vi "Set Impulse Data.vi"(8 "error in (no error)":errorcluster, 10 "Impulse Object Reference":T1, 11 "Impulse Manager in":refnum<class "Impulse Manager.lvclass">) -> (0 "error out":errorcluster, 3 "Impulse Manager out":refnum<class "Impulse Manager.lvclass">)   [LabVIEW 2016, in "Impulse Manager.lvclass"]
uses:
  Impulse Manager.lvclass
  Impulse Data/Instance handle.ctl
  Impulse Data/Impulse Data.lvclass
  Impulse Manager.lvclass/Impulse Manager.ctl
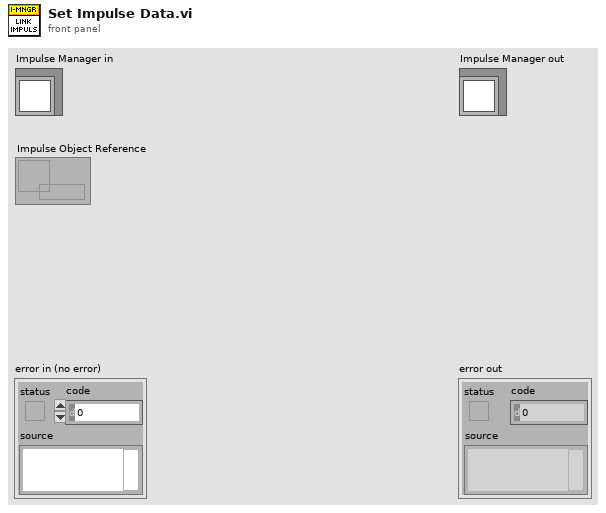
[diagram p1: front panel]
types:
  T1 = typedef "Impulse Data.lvclass/Instance handle.ctl" = refnum<data-value>
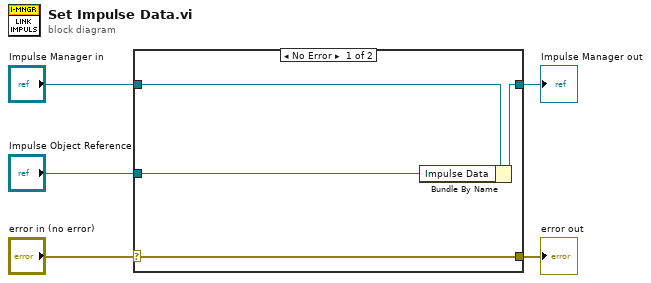
[diagram p0: block diagram]
diagram:
  n1 = case shown="No Error" "error in (no error)" {
    selector: "error in (no error)" -> [w9 w10]
    tunnel: [w9 w10] -> w4
    tunnel: [w7 w11] -> w2
    tunnel: "Impulse Manager in" -> [w8 w11]
    tunnel: "Impulse Object Reference" -> [w6 _]
    frame No Error {
      n2 = Bundle By Name(cluster=w8, "Impulse Data"=w6) -> (w7:refnum<class "Impulse Manager.lvclass">)
    }
    frame Error {
    }
  }
  "error out" <- w4
  "Impulse Manager out" <- w2
